vi "angle setpoint.vi"(8 "kp":dbl, 9 "angle to point":dbl, 10 "theta desired":dbl, 11 "distance":dbl) -> (3 "angle setpoint":dbl)   [LabVIEW 2015]
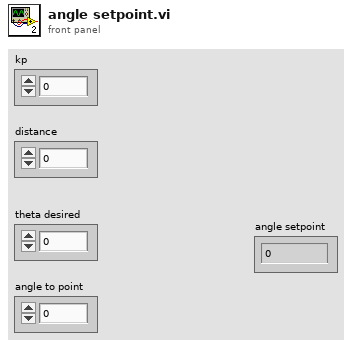
[diagram p1: front panel]
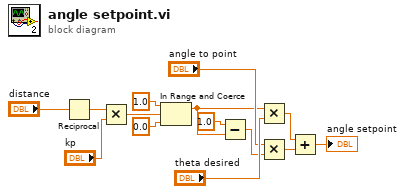
[diagram p0: block diagram]
diagram:
  n1 = Reciprocal(x="distance") -> (1/x=w3:dbl)
  n2 = Multiply(x=w3, y="kp") -> (x*y=w1:dbl)
  n3 = In Range and Coerce(upper limit=1.0, x=w1, lower limit=0.0) -> (coerced(x)=w5:dbl)  [unwired: 1 out]
  n4 = Subtract(x=1.0, y=w5) -> (x-y=w9:dbl)
  n5 = Multiply(x=w5, y="theta desired") -> (x*y=w8:dbl)
  n6 = Multiply(x="angle to point", y=w9) -> (x*y=w7:dbl)
  n7 = Add(x=w8, y=w7) -> (x+y=→"angle setpoint":dbl)
